vi "debugger.vi"(7 "httpRequestID":u32) -> ()   [LabVIEW 2011]
doc: "This VI is a state machine that can be ran from a Browser."
uses:
  server/database/Users/User Record.ctl
  <vilib>/wsapi/NI_WebServices.lvlib
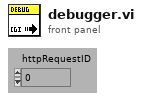
[diagram p1: front panel]
types:
  T1 = typedef "User Record.ctl" = cluster{"ixUser":i32, "sxUsername":string, "sLastName":string, "sFirstName":string, "sEmail":string, "sPassword":string, "tLoginTime":timestamp, "sLoginComputer":string, "fAdministrator":bool, "fRunSequences":bool, "fModifySequences":bool, "fRunScenarios":bool, "fModifyScenarios":bool, "fModifyTemplates":bool, "fModifyUsers":bool, "fModifyStations":bool, "fModifyFields":bool}
  T2 = typedef "Connection Refnum.ctl" = cluster{"Environment Handle":i32, "Connection Handle":i32}
  T3 = typedef "Keyed Array.ctl" = cluster{"keys":string[], "values":string[]}
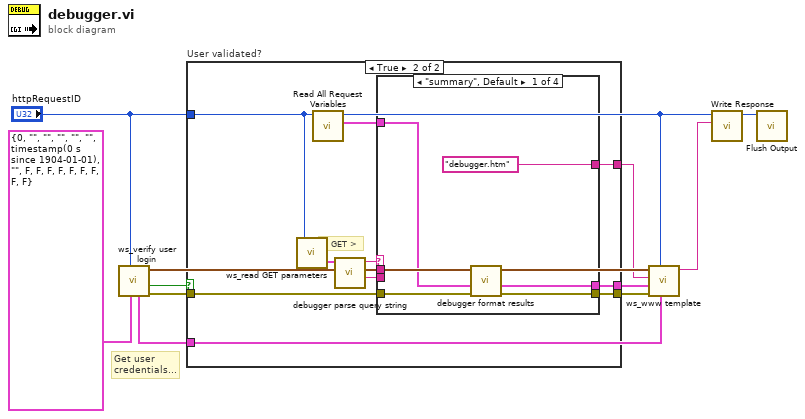
[diagram p0: block diagram]
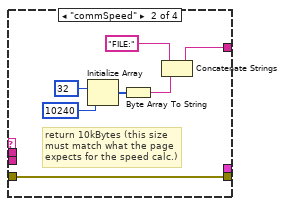
[diagram p3: hidden frame]
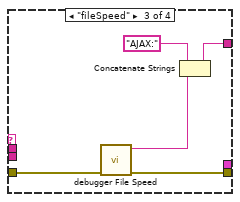
[diagram p4: hidden frame]
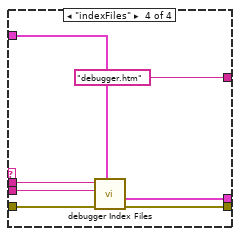
[diagram p5: hidden frame]
diagram:
  # "Get user \ncredentials..."
  n1 = call "ws_verify user login.vi"("Required Permisions"=T1 {"ixUser"=0, "sxUsername"="", "sLastName"="", "sFirstName"="", "sEmail"="", "sPassword"="", "tLoginTime"=timestamp(0 s since 1904-01-01), "sLoginComputer"="", "fAdministrator"=FALSE, "fRunSequences"=FALSE, "fModifySequences"=FALSE, "fRunScenarios"=FALSE, "fModifyScenarios"=FALSE, "fModifyTemplates"=FALSE, "fModifyUsers"=FALSE, "fModifyStations"=FALSE, "fModifyFields"=FALSE} ("User Record"), "httpRequestID"="httpRequestID") -> ("error out"=w10:errorcluster, "User Verified\nand Spartan\nAuthorized?"=w11:bool, "DB Connection Ref"=w7:T2, "User"=w4:T1)  [unwired: 6 in]
  n2 = case "User validated?" shown="True" w11 {
    tunnel: w10 -> [w12 w17]
    tunnel: [w12 w18] -> w8
    tunnel: [_ w13] -> w5
    tunnel: [_ w14] -> w6
    tunnel: w4 -> [_ _]
    tunnel: "httpRequestID" -> [_ w22]
    frame False {
    }
    frame True {
      # "< GET >"
      n3 = call "ws_read GET parameters.vi"("httpRequestID"=w22) -> ("GET query params"=w16:T3)  [unwired: 2 in]
      n4 = call <vilib>:"Read All Request Variables.vi"("httpRequestID"=w22) -> ("request variables"=w15:cluster{"Key":string[], "Value":string[]})  [unwired: 8 in, 2 out]
      n5 = call "debugger parse query string.vi"("ENV"=w16) -> ("Serial Number"=w21:string, "Model Number"=w20:string, "Action"=w19:string)  [unwired: 8 in]
      n6 = case shown="\"summary\", Default" w19 {
        tunnel: [w26 w34 w38 w44] -> w18
        tunnel: w17 -> [w27 w34 w39 w45]
        tunnel: [w25 _ _ w41] -> w14
        tunnel: ["debugger.htm" w29 w37 "debugger.htm"] -> w13
        tunnel: w15 -> [w23 _ _ w40]
        tunnel: w20 -> [_ _ _ w43]
        tunnel: w21 -> [_ _ _ w42]
        frame "summary", Default {
          n7 = call "debugger format results.vi"("error in (no error)"=w27, "ENV"=w23) -> ("error out"=w26:errorcluster, "Template Keys"=w25:T3)  [unwired: 3 in, 5 out]
        }
        frame "commSpeed" {
          # "return 10kBytes (this size\nmust match what the page\nexpects for the speed calc.)"
          n8 = Initialize Array(u8 32, 10240 ("dimension size")) -> (w31:u8[])
          n9 = Byte Array To String(unsigned byte array=w31) -> (string=w28:string)
          n10 = Concatenate Strings("FILE:", w28) -> (w29:string)
        }
        frame "fileSpeed" {
          n11 = call "debugger File Speed.vi"("error in (no error)"=w39) -> ("error out"=w38:errorcluster, "js timing results"=w35:string)  [unwired: 3 in, 6 out]
          n12 = Concatenate Strings("AJAX:", w35) -> (w37:string)
        }
        frame "indexFiles" {
          n13 = call "debugger Index Files.vi"("ENV"=w40, "error in (no error)"=w45, "Serial Number"=w42, "Model Number"=w43) -> ("error out"=w44:errorcluster, "Template Keys"=w41:T3)  [unwired: 6 in]
        }
      }
    }
  }
  n14 = call "ws_www template.vi"("User"=w4, "httpRequestID"="httpRequestID", "error in (no error)"=w8, "Template Keys (empty)"=w6, "Template (\"\")"=w5, "DB Connection Ref"=w7) -> ("HTTP Template Content"=w2:string)  [unwired: 5 in]
  n15 = call <vilib>:"Write Response.vi"("response string"=w2, "httpRequestID"="httpRequestID") -> ("httpRequestID out"=w3:u32)  [unwired: 8 in, 1 out]
  n16 = call <vilib>:"Flush Output.vi"("httpRequestID"=w3) -> ()  [unwired: 9 in, 2 out]
